vi "Configure Output Phase.vi"(8 "error in (no error)":errorcluster, 9 "Output Phase (0.0 degrees)":dbl min=0.0 max=359.7 format="%.1f", 10 "Output Sync (0: Immediate)":i32(ring) items=["Immediate", "Phase"], 11 "VISA resource name":refnum<visa-resource-name>) -> (0 "error out":errorcluster, 3 "VISA resource name out":refnum<visa-resource-name>)   [LabVIEW 2015, in "BK Precision 983X Series.lvlib"]
doc: "Configures the output sync and phase."
uses:
  <instrlib>/BK Precision 983X Series/BK Precision 983X Series.lvlib
panel:
  # "degree"
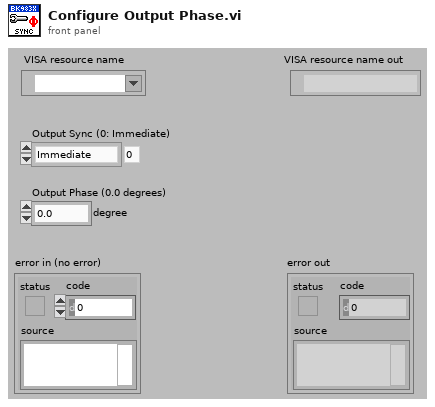
[diagram p1: front panel]
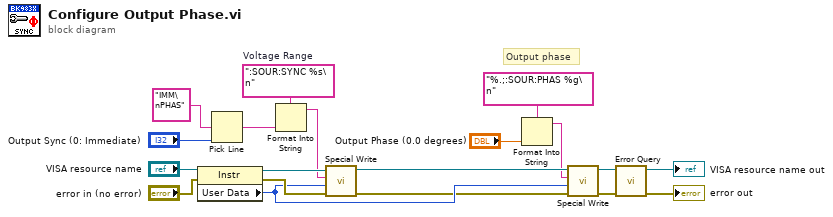
[diagram p0: block diagram]
diagram:
  w3 = ":SOUR:SYNC %s\n"  # Voltage Range
  # "Output phase"
  n1 = property class="Instr"(reference="VISA resource name", error in="error in (no error)") -> (reference out=w14:refnum<visa-resource-name>, error out=w15:errorcluster, "User Data"=w5:u32)
  n2 = Pick Line(multi-line string="IMM\nPHAS", line index="Output Sync (0: Immediate)") -> (output string=w2:string)  [unwired: 1 in]
  n3 = Format Into String(format string=w3, w2) -> (resulting string=w1:string)  [unwired: 2 in, 1 out]
  n4 = call <instrlib>:"Special Write.vi"("error in (no error)"=w15, "Delay (0 ms)"=w5, "Input String"=w1, "VISA resource name"=w14) -> ("error out"=w4:errorcluster, "VISA resource name out"=w7:refnum<visa-resource-name>)  [unwired: 6 in]
  n5 = Format Into String(format string="%.;:SOUR:PHAS %g\n", "Output Phase (0.0 degrees)") -> (resulting string=w6:string)  [unwired: 2 in, 1 out]
  n6 = call <instrlib>:"Special Write.vi"("error in (no error)"=w4, "Delay (0 ms)"=w5, "Input String"=w6, "VISA resource name"=w7) -> ("error out"=w8:errorcluster, "VISA resource name out"=w9:refnum<visa-resource-name>)  [unwired: 6 in]
  n7 = call <instrlib>:"Error Query.vi"("error in (no error)"=w8, "VISA resource name"=w9) -> ("error out"=→"error out":errorcluster, "VISA resource name out"=→"VISA resource name out":refnum<visa-resource-name>)  [unwired: 6 in, 2 out]
